vi "FMDLCloseKeithley2450.vi"(1 "error in (no error)":errorcluster, 2 "VISA resource name":refnum<visa-resource-name>) -> (0 "error out":errorcluster)   [LabVIEW 2018]
uses:
  <instrlib>/Keithley 2450/Keithley 2450.lvlib
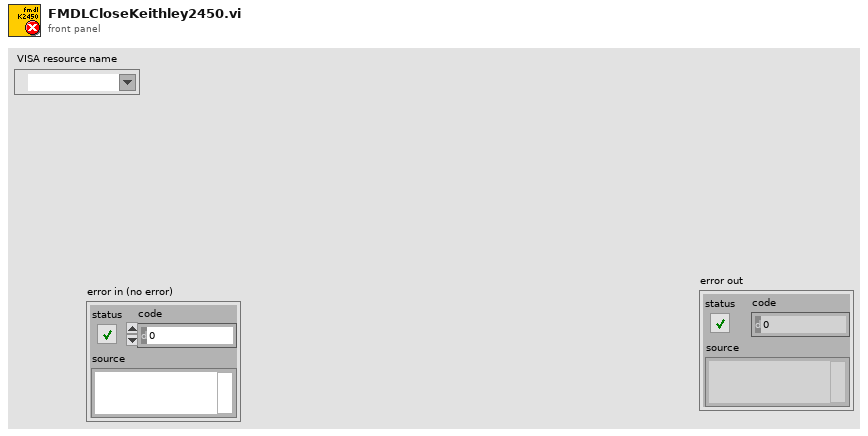
[diagram p1: front panel]
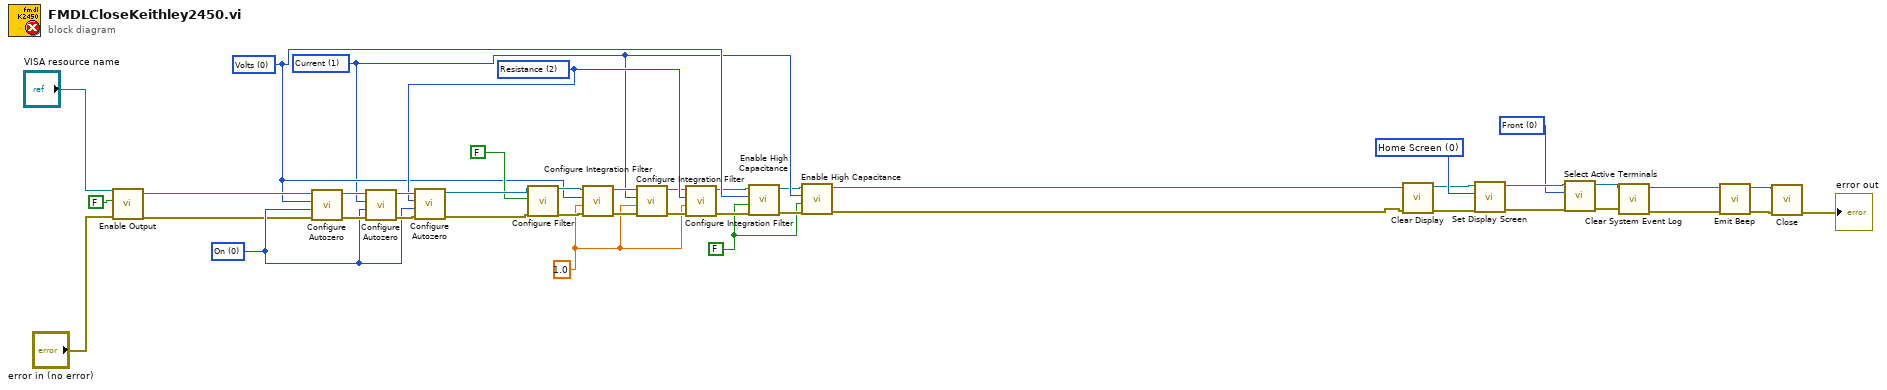
[diagram p0: block diagram]
diagram:
  w5 = u16 0 items=["Front", "Rear"] ("Active Terminals (0: Front)")
  w14 = u16 0 items=["Home Screen", "Source Screen", "Plot Screen", "User-defined Screen", "Statistics Screen", "Settings Screen", "Graph Screen", "Data sheet Screen"] ("Screen Home")
  w15 = FALSE ("Enable High Capacitance (T:Enable)")
  w22 = 1.0 ("Measurement Speed (1 PLC)")
  w25 = u16 2 items=["Volts", "Current", "Resistance"] ("Function (0: Volts)")
  w20 = u16 1 items=["Volts", "Current", "Resistance"] ("Function (0: Volts)")
  w39 = u16 0 items=["On", "Off"] ("Autozero  (0: On)")
  w21 = u16 0 items=["Volts", "Current", "Resistance"] ("Function (0: Volts)")
  n1 = call <instrlib>:"Enable Output.vi"("error in (no error)"="error in (no error)", "Enable Output (T: Enable)"=FALSE, "VISA resource name"="VISA resource name") -> ("error out"=w33:errorcluster, "VISA resource name out"=w35:refnum<visa-resource-name>)  [unwired: 7 in]
  n2 = call <instrlib>:"Configure Autozero.vi"("error in (no error)"=w33, "Autozero  (0: On)"=w39, "Function (0: Volts)"=w21, "VISA resource name"=w35) -> ("error out"=w42:errorcluster, "VISA resource name out"=w43:refnum<visa-resource-name>)  [unwired: 6 in]
  n3 = call <instrlib>:"Configure Autozero.vi"("error in (no error)"=w42, "Autozero  (0: On)"=w39, "Function (0: Volts)"=w20, "VISA resource name"=w43) -> ("error out"=w40:errorcluster, "VISA resource name out"=w41:refnum<visa-resource-name>)  [unwired: 6 in]
  n4 = call <instrlib>:"Configure Autozero.vi"("error in (no error)"=w40, "Autozero  (0: On)"=w39, "Function (0: Volts)"=w25, "VISA resource name"=w41) -> ("error out"=w31:errorcluster, "VISA resource name out"=w32:refnum<visa-resource-name>)  [unwired: 6 in]
  n5 = call <instrlib>:"Configure Filter.vi"("VISA resource name"=w32, "Enable Filter  (T: Enable)"=FALSE, "error in (no error)"=w31) -> ("VISA resource name out"=w29:refnum<visa-resource-name>, "error out"=w28:errorcluster)  [unwired: 15 in]
  n6 = call <instrlib>:"Configure Integration Filter.vi"("error in (no error)"=w28, "Measurement Speed (1 PLC)"=w22, "Function (0: Volts)"=w21, "VISA resource name"=w29) -> ("error out"=w26:errorcluster, "VISA resource name out"=w27:refnum<visa-resource-name>)  [unwired: 6 in]
  n7 = call <instrlib>:"Configure Integration Filter.vi"("error in (no error)"=w26, "Measurement Speed (1 PLC)"=w22, "Function (0: Volts)"=w20, "VISA resource name"=w27) -> ("error out"=w23:errorcluster, "VISA resource name out"=w24:refnum<visa-resource-name>)  [unwired: 6 in]
  n8 = call <instrlib>:"Configure Integration Filter.vi"("error in (no error)"=w23, "Measurement Speed (1 PLC)"=w22, "Function (0: Volts)"=w25, "VISA resource name"=w24) -> ("error out"=w18:errorcluster, "VISA resource name out"=w19:refnum<visa-resource-name>)  [unwired: 6 in]
  n9 = call <instrlib>:"Enable High Capacitance.vi"("error in (no error)"=w18, "Enable High Capacitance (T:Enable)"=w15, "Function (0: Volts)"=w21, "VISA resource name"=w19) -> ("error out"=w16:errorcluster, "VISA resource name out"=w17:refnum<visa-resource-name>)  [unwired: 6 in]
  n10 = call <instrlib>:"Enable High Capacitance.vi"("error in (no error)"=w16, "Enable High Capacitance (T:Enable)"=w15, "Function (0: Volts)"=w20, "VISA resource name"=w17) -> ("error out"=w1:errorcluster, "VISA resource name out"=w2:refnum<visa-resource-name>)  [unwired: 6 in]
  n11 = call <instrlib>:"Clear Display.vi"("error in (no error)"=w1, "VISA resource name"=w2) -> ("error out"=w3:errorcluster, "VISA resource name out"=w4:refnum<visa-resource-name>)  [unwired: 8 in]
  n12 = call <instrlib>:"Set Display Screen.vi"("error in (no error)"=w3, "Screen Home"=w14, "VISA resource name"=w4) -> ("error out"=w6:errorcluster, "VISA resource name out"=w7:refnum<visa-resource-name>)  [unwired: 7 in]
  n13 = call <instrlib>:"Select Active Terminals.vi"("error in (no error)"=w6, "Active Terminals (0: Front)"=w5, "VISA resource name"=w7) -> ("error out"=w8:errorcluster, "VISA resource name out"=w9:refnum<visa-resource-name>)  [unwired: 7 in]
  n14 = call <instrlib>:"Clear System Event Log.vi"("error in (no error)"=w8, "VISA resource name"=w9) -> ("error out"=w10:errorcluster, "VISA resource name out"=w11:refnum<visa-resource-name>)  [unwired: 8 in]
  n15 = call <instrlib>:"Emit Beep.vi"("error in (no error)"=w10, "VISA resource name"=w11) -> ("error out"=w13:errorcluster, "VISA resource name out"=w12:refnum<visa-resource-name>)  [unwired: 8 in]
  n16 = call <instrlib>:"Close.vi"("error in (no error)"=w13, "VISA resource name"=w12) -> ("error out"=→"error out":errorcluster)  [unwired: 9 in]
